vi "Gets Target Data Array.vi"(8 "error in (no error)":errorcluster) -> (0 "error out":errorcluster, 3 "All Targets Data":T1(array[cluster]))   [LabVIEW 2014]
doc: "Gets the IP and OS of each target in the active system definition"
uses:
  NationalInstruments.VeriStand.SystemDefinitionAPI
  <vilib>/NI Veristand/Custom Device Tools/Custom Device Utility Library/Custom Device Utility Library.lvlib
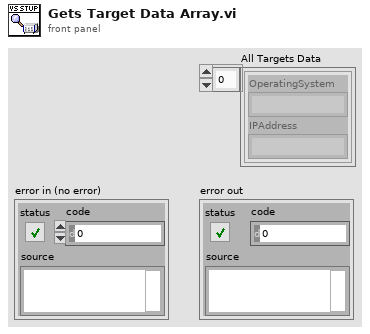
[diagram p1: front panel]
types:
  T1 = cluster{"OperatingSystem":string, "IPAddress":string}[]
  T2 = cluster{"OperatingSystem":string, "IPAddress":string}
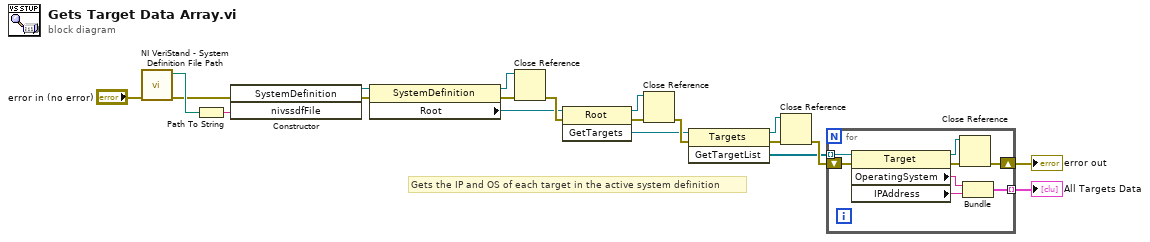
[diagram p0: block diagram]
diagram:
  # "Gets the IP and OS of each target in the active system definition"
  n1 = call <vilib>:"NI VeriStand - System Definition File Path.vi"("error in (no error)"="error in (no error)") -> ("error out"=w2:errorcluster, "SDF path"=w4:path)  [unwired: 9 in]
  n2 = Path To String(path=w4) -> (string=w3:string)
  n3 = constructor class="SystemDefinition"(error in=w2, "nivssdfFile"=w3) -> (reference out=w5:refnum<k24>, error out=w6:errorcluster)  [unwired: 2 in, 2 out]
  n4 = property class="SystemDefinition"(reference=w5, error in=w6) -> (reference out=w11:refnum<k24>, error out=w10:errorcluster, "Root"=w7:refnum<k24>)
  n5 = Close Reference(reference=w11, error in (no error)=w10) -> (error out=w12:errorcluster)
  n6 = invoke class="Root" method="GetTargets"(reference=w7, error in=w12) -> (reference out=w14:refnum<k24>, error out=w13:errorcluster, "GetTargets"=w8:refnum<k24>)  [unwired: 1 in]
  n7 = Close Reference(reference=w14, error in (no error)=w13) -> (error out=w15:errorcluster)
  n8 = invoke class="Targets" method="GetTargetList"(reference=w8, error in=w15) -> (reference out=w17:refnum<k24>, error out=w16:errorcluster, "GetTargetList"=w9:refnum<k24>[])  [unwired: 1 in]
  n9 = Close Reference(reference=w17, error in (no error)=w16) -> (error out=w18:errorcluster)
  n10 = for {
    tunnel: w9 -> [w28] mode=indexing
    shift-right: [w26] -> w20
    shift-left: w18 -> [w27]
    tunnel: [w21] -> w19 mode=indexing
    n11 = property class="Target"(reference=w28, error in=w27) -> (reference out=w24:refnum<k24>, error out=w25:errorcluster, "OperatingSystem"=w23:string, "IPAddress"=w22:string)
    n12 = Close Reference(reference=w24, error in (no error)=w25) -> (error out=w26:errorcluster)
    n13 = Bundle("OperatingSystem"=w23, "IPAddress"=w22) -> (w21:T2)  [unwired: 1 in]
  }
  "error out" <- w20
  "All Targets Data" <- w19
